vi "Finish.vi"   [LabVIEW 2014]
doc: "This VI is called just before exiting. It is expected to close I/O refnum, save collected data, etc."
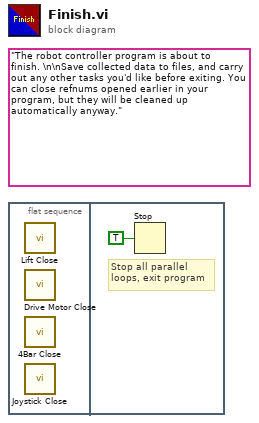
[diagram p0: block diagram]
diagram:
  (unwired) "The robot controller program is about to finish. \n\nSave collected data to files, and carry out any other tasks you'd like before exiting. You can close refnums opened earlier in your program, but they will be cleaned up automatically anyway."
  n1 = flat-sequence {
    frame #0 {
      n2 = call "Lift Close.vi"() -> ()  [unwired: 1 in, 1 out]
      n3 = call "Drive Motor Close.vi"() -> ()  [unwired: 1 in, 1 out]
      n4 = call "4Bar Close.vi"() -> ()  [unwired: 1 in, 1 out]
      n5 = call "Joystick Close.vi"() -> ()  [unwired: 12 in]
    }
    frame #1 {
      # "Stop all parallel\nloops, exit program"
      n6 = Stop(stop? (T)=TRUE ("Quit")) -> ()
    }
  }
